vi "XIPIN_LDPC_802_16_Encoder_1_0.vi"   [LabVIEW 2017]
doc: "The Xilinx 802.16e Low Density Parity Check code Encoder LogiCORE is a drop in module for Virtex-II(TM), Virtex-4(TM) and Spartan-3(TM) families of FPGA. It is a high-speed, compact module for generating data streams according to the IEEE 802.16e-2005 (draft 6) standard, OFDMA PHY layer. (Section 8.4.9.2.5) The core is fully synchronous, using a single clock, and integrates seamlessly with the Xilinx design flow.\n------------------------------------\n<b>Need License</b> : Yes"
uses:
  <vilib>/rvi/XilinxIP/XIPIN_XNode/niFpgaXIPIN.xnode
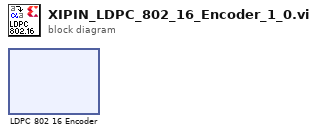
[diagram p0: block diagram]
diagram:
  n1 = xnode ("LDPC 802 16 Encoder")() -> ()
